vi "pc_fit_2_gauss.vi"(6 "error in (no error)":errorcluster, 8 "peak offset":dbl=0.00075, 9 "Center requested peak":dbl, 10 "Y-Data":dbl[](array[numeric]), 11 "X-Data":dbl[](array[numeric])) -> (1 "residue":dbl, 2 "fit coeff":T1, 3 "best nonlinear fit":dbl[](array[numeric]), 4 "error out":errorcluster)   [LabVIEW 2018, in "Plots.lvclass"]
doc: "the vi tries to fit two gauss functions.\nOutput are the peak parameters and the best fit values"
uses:
  Plots.lvclass
  <vilib>/gmath/NumericalOptimization/Nonlinear Curve Fit LM formula string.vi
  <vilib>/gmath/NI_Gmath.lvlib
panel:
  out "XY Graph":cluster{cluster{dbl, "Numeric":dbl}[]}[](graph)
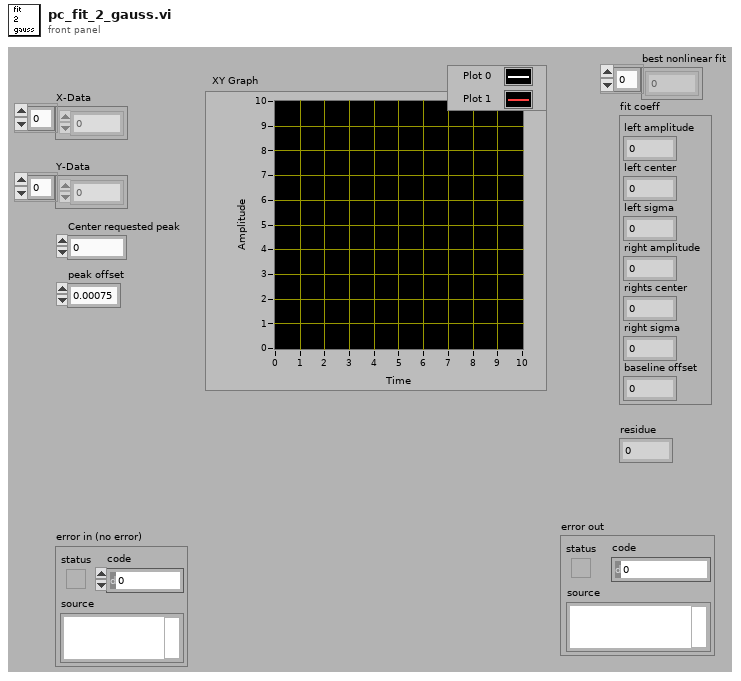
[diagram p1: front panel]
types:
  T1 = cluster{"left amplitude":dbl, "left center":dbl, "left sigma":dbl, "right amplitude":dbl, "rights center":dbl, "right sigma":dbl, "baseline offset":dbl}
  T2 = cluster{"model":string, "Parameters":string[], "x":string}
  T3 = cluster{"Numeric":dbl, "Numeric":dbl, "Numeric":dbl, "Numeric":dbl, "Numeric":dbl, "Numeric":dbl, "Numeric":dbl}
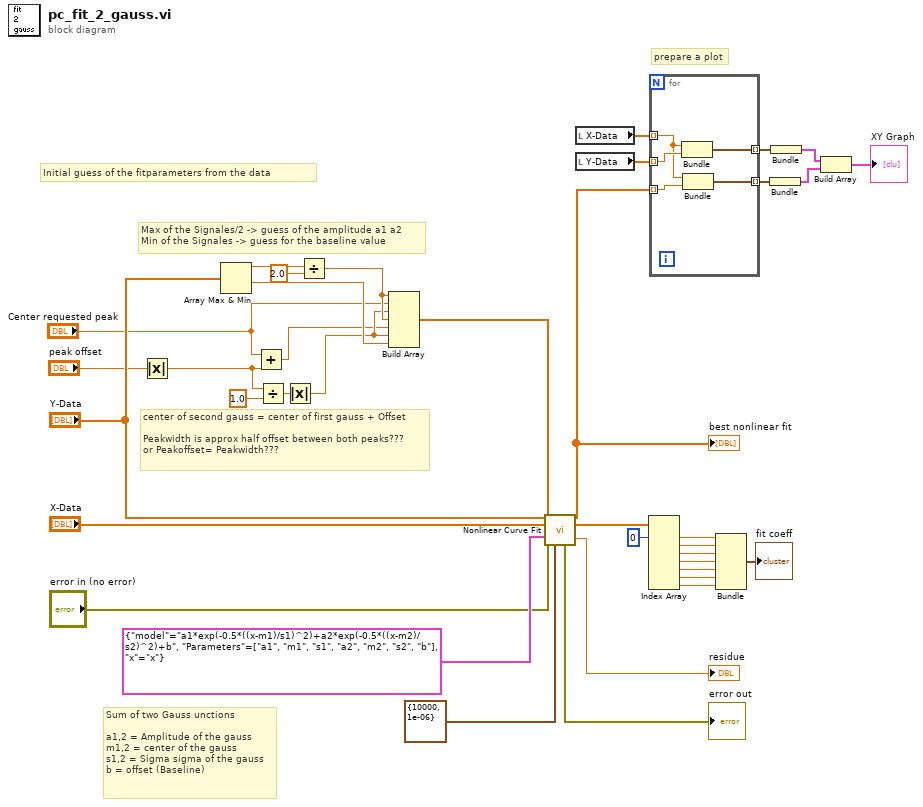
[diagram p0: block diagram]
diagram:
  # "prepare a plot"
  # "Sum of two Gauss unctions\n\na1,2 = Amplitude of the gauss\nm1,2 = center of the gauss\ns1,2 = Sigma sigma of the gauss\nb = offset (Baseline)"
  # "center of second gauss = center of first gauss + Offset\n\nPeakwidth is approx half offset between both peaks???\nor Peakoffset= Peakwidth???"
  # "Max of the Signales/2 -> guess of the amplitude a1 a2\nMin of the Signales -> guess for the baseline value"
  # "Initial guess of the fitparameters from the data"
  n1 = Absolute Value(x="peak offset") -> (abs(x)=w9:dbl)
  n2 = Array Max & Min(array="Y-Data") -> (max value=w32:dbl, min value=w29:dbl)  [unwired: 2 out]
  n3 = Add(x="Center requested peak", y=w9) -> (x+y=w11:dbl)
  n4 = Divide(x=w9, y=1.0) -> (x/y=w14:dbl)
  n5 = Absolute Value(x=w14) -> (abs(x)=w13:dbl)
  n6 = Divide(x=w32, y=2.0) -> (x/y=w34:dbl)
  n7 = Build Array(w34, "Center requested peak", w13, w34, w11, w13, w29) -> (w30:dbl[])
  n8 = call-poly <vilib>:"Nonlinear Curve Fit.vi"("Y"="Y-Data", "initial parameters"=w30, "X"="X-Data", "model description"=T2 {"model"="a1*exp(-0.5*((x-m1)/s1)^2)+a2*exp(-0.5*((x-m2)/s2)^2)+b", "Parameters"=["a1", "m1", "s1", "a2", "m2", "s2", "b"], "x"="x"}, "error in (no error)"="error in (no error)", "termination"=cluster{"max iteration":i32, "tolerance":dbl} {"max iteration"=10000, "tolerance"=1e-06}) -> ("best nonlinear fit"=w6:dbl[], "best fit parameters"=w24:dbl[], "residue"=→"residue":dbl, "error out"=→"error out":errorcluster)  [unwired: 5 in, 1 out]
  "best nonlinear fit" <- w6
  n9 = local read "X-Data"() -> (w8:dbl[])
  n10 = local read "Y-Data"() -> (w7:dbl[])
  n11 = Index Array(array=w24, index #1=0 ("index")) -> (element #1=w23:dbl, element #2=w22:dbl, element #3=w21:dbl, element #4=w20:dbl, element #5=w19:dbl, element #6=w18:dbl, element #7=w17:dbl)  [unwired: 6 in]
  n12 = for {
    tunnel: w8 -> [w40] mode=indexing
    tunnel: w7 -> [w42] mode=indexing
    tunnel: w6 -> [w41] mode=indexing
    tunnel: [w39] -> w5 mode=indexing
    tunnel: [w38] -> w4 mode=indexing
    n13 = Bundle(w40, w42) -> (w39:cluster{dbl, dbl})  [unwired: 1 in]
    n14 = Bundle(w40, "Numeric"=w41) -> (w38:cluster{dbl, "Numeric":dbl})  [unwired: 1 in]
  }
  n15 = Bundle("Numeric"=w23, "Numeric"=w22, "Numeric"=w21, "Numeric"=w20, "Numeric"=w19, "Numeric"=w18, "Numeric"=w17) -> (→"fit coeff":T3)  [unwired: 1 in]
  n16 = Bundle(w4) -> (w2:cluster{cluster{dbl, "Numeric":dbl}[]})  [unwired: 1 in]
  n17 = Bundle(w5) -> (w3:cluster{cluster{dbl, dbl}[]})  [unwired: 1 in]
  n18 = Build Array(w3, w2) -> (→"XY Graph":cluster{cluster{dbl, "Numeric":dbl}[]}[])
